vi "simplePID_FXP_integralsatfixed.vi"(0 "setpoint":fxp<+/-,16,10>, 1 "reset? (F)":bool, 2 "Input Selector":u16, 3 "channel (0)":u16, 5 "process variable":fxp<+/-,16,10>, 7 "manual control":T3, 12 "Gains":T1, 13 "output range":T5={"output high (Inf)"=2047.99609375, "output low (-Inf)"=-2048.0}, 14 "setpoint weighting":T4={"proportional weighting (1)"=1.0, "derivative weighting (0)"=0.0}) -> (4 "output":fxp<+/-,20,12> format="%.12g", 6 "error":fxp<+/-,16,10> format="%.11g", 8 "actions":T2)   [LabVIEW 2020]
uses:
  Typedef/niFpgaPID_OutputRange_FXP.ctl
  Typedef/niFpgaPID_SetpointWeightings_FXP.ctl
  Typedef/niFpgaPID_ManualControl_FXP.ctl
  Typedef/niFpgaPID_PIDActions_FXP.ctl
  Typedef/niFpgaPID_PIDGains_FXP.ctl
  Typedef/niFpgaPID_PIDErrors_FXP.ctl
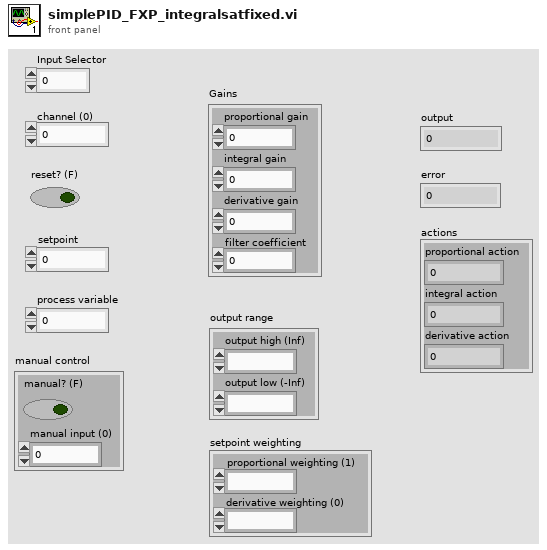
[diagram p1: front panel]
types:
  T1 = typedef "niFpgaPID_PIDGains_FXP.ctl" = cluster{"proportional gain":fxp<+/-,17,4>, "integral gain":fxp<+/-,16,3>, "derivative gain":fxp<+/-,16,3>, "filter coefficient":fxp<+/-,17,4>}
  T2 = typedef "niFpgaPID_PIDActions_FXP.ctl" = cluster{"proportional action":fxp<+/-,20,12>, "integral action":fxp<+/-,20,12>, "derivative action":fxp<+/-,20,12>}
  T3 = typedef "niFpgaPID_ManualControl_FXP.ctl" = cluster{"manual? (F)":bool, "manual input (0)":fxp<+/-,20,12>}
  T4 = typedef "niFpgaPID_SetpointWeightings_FXP.ctl" = cluster{"proportional weighting (1)":fxp<+/-,16,2>, "derivative weighting (0)":fxp<+/-,16,2>}
  T5 = typedef "niFpgaPID_OutputRange_FXP.ctl" = cluster{"output high (Inf)":fxp<+/-,20,12>, "output low (-Inf)":fxp<+/-,20,12>}
  T6 = typedef "niFpgaPID_PIDErrors_FXP.ctl" = cluster{"error":fxp<+/-,16,10>, "error with beta":fxp<+/-,16,10>, "error with gamma":fxp<+/-,16,10>}
  T7 = typedef "niFpgaPID_PIDState_FXP.ctl" = cluster{"uI(k-1)":fxp<+/-,20,12>, "e(k-1)":fxp<+/-,16,10>, "e(k-1) with gamma":fxp<+/-,16,10>, "uD(k-1)":fxp<+/-,20,12>}
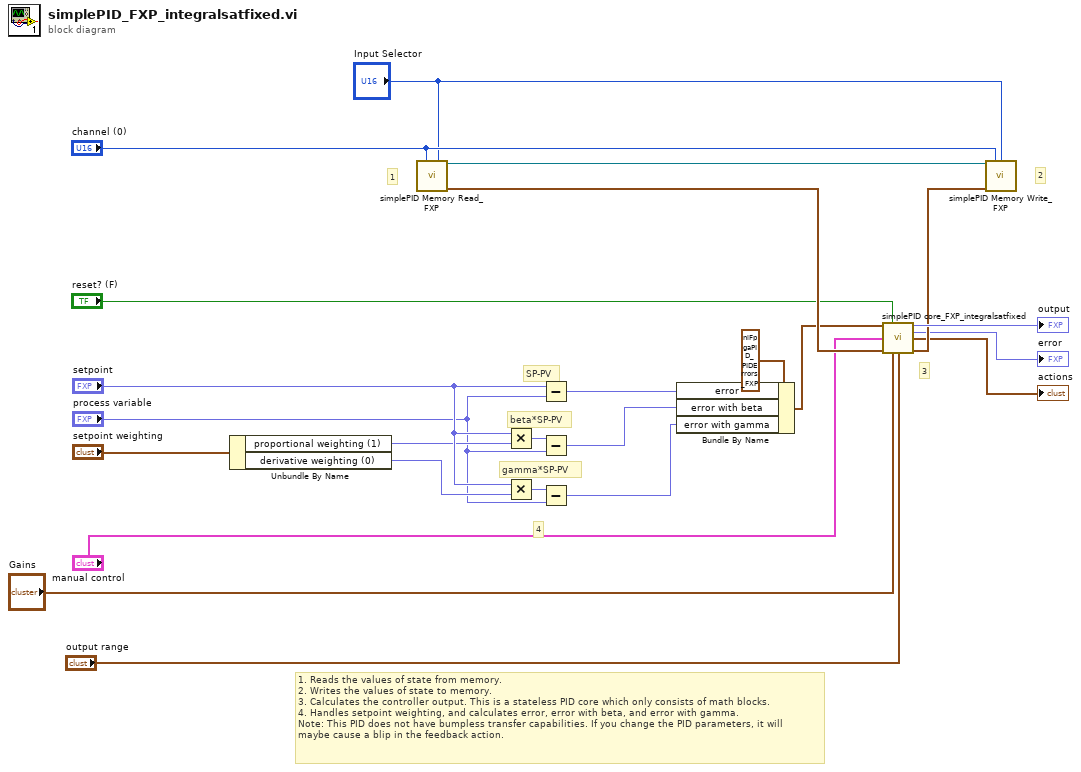
[diagram p0: block diagram]
diagram:
  # "SP-PV"
  # "beta*SP-PV"
  # "gamma*SP-PV"
  # "1. Reads the values of state from memory.\n2. Writes the values of state to memory.\n3. Calculates the controller output. This is a stateless PID core which only consists of math blocks.\n4. Handles setpoint weighting, and calculates error, error with beta, and error with gamma.\nNote: This PID does not have bumpless transfer capabilities. If you change the PID parameters, it will\nmaybe cause a blip in the feedback action."
  # "4"
  # "3"
  # "2"
  # "1"
  n1 = Unbundle By Name("setpoint weighting") -> ("proportional weighting (1)"=w16:fxp<+/-,16,2>, "derivative weighting (0)"=w22:fxp<+/-,16,2>)
  n2 = call "simplePID Memory Read_FXP.vi"("channel (0)"="channel (0)", "Input Selector"="Input Selector") -> ("Memory Out"=w2:refnum<k21>, "state out"=w20:T7)  [unwired: 12 in]
  n3 = Multiply(x="setpoint", y=w16) -> (x*y=w4:fxp<+/-,16,10>)
  n4 = Multiply(x="setpoint", y=w22) -> (x*y=w5:fxp<+/-,16,10>)
  n5 = Subtract(x="setpoint", y="process variable") -> (x-y=w8:fxp<+/-,16,10>)
  n6 = Subtract(x=w4, y="process variable") -> (x-y=w13:fxp<+/-,16,10>)
  n7 = Subtract(x=w5, y="process variable") -> (x-y=w12:fxp<+/-,16,10>)
  n8 = Bundle By Name(cluster=T6 {"error"=0.0, "error with beta"=0.0, "error with gamma"=0.0} ("errors"), "error"=w8, "error with beta"=w13, "error with gamma"=w12) -> (w11:T6)
  n9 = call "simplePID core_FXP_integralsatfixed.vi"("errors"=w11, "reset? (F)"="reset? (F)", "manual control"="manual control", "state in"=w20, "gains"="Gains", "output range"="output range") -> ("output"=→"output":fxp<+/-,20,12>, "error"=→"error":fxp<+/-,16,10>, "actions"=→"actions":T2, "state out"=w21:T7)  [unwired: 6 in]
  n10 = call "simplePID Memory Write_FXP.vi"("Memory In"=w2, "channel (0)"="channel (0)", "Input Selector"="Input Selector", "state in"=w21) -> ()  [unwired: 12 in]
